vi "Actor Core.vi"(8 "error in":errorcluster, 11 "CS++Motor in":refnum<class "CS++Motor.lvclass">) -> (0 "error out":errorcluster, 3 "Actor out":refnum<class "Actor.lvclass">)   [LabVIEW 2015, in "CS++Motor.lvlib" / "CS++Motor.lvclass"]
doc: "(<B>Filename</B>: Actor Framework.lvlib:Actor.lvclass:Actor Core.vi)\n\nReceives messages to the actor, reacts to them, and initiates any error handling that may shut the actor down.\n\nDescendant classes may override this VI to append parallel tasks for the actor to complete while it handles messages. Overrides use the Call Parent Method node."
uses:
  CS++Motor.lvclass
  <vilib>/ActorFramework/Actor/Actor.lvclass
  CS++Motor.lvclass/CS++Motor.ctl
  <vilib>/ActorFramework/Message Enqueuer/Message Priority.ctl
  <vilib>/ActorFramework/Actor/Actor.lvclass/Actor.ctl
  <vilib>/ActorFramework/Message Enqueuer/Message Enqueuer.lvclass/Message Enqueuer.ctl
  <vilib>/ActorFramework/Report Error Msg/Report Error Msg.lvclass/Report Error Msg.ctl
  <vilib>/ActorFramework/Message Enqueuer/Init from Existing Queue.vi
  <vilib>/ActorFramework/Message Enqueuer/Enqueue.vi
  <vilib>/ActorFramework/Message Priority Queue/Priority Enqueue.vi
  CSPP_Core/Actors/CS++DeviceActor/CS++DeviceActor.lvclass
  <vilib>/ActorFramework/Message Enqueuer/Message Enqueuer.lvclass
  <vilib>/ActorFramework/Report Error Msg/Report Error Msg.lvclass
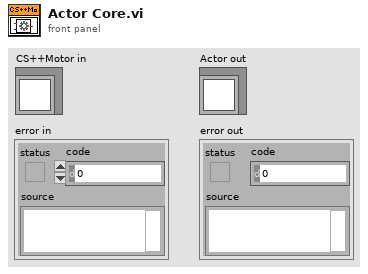
[diagram p1: front panel]
types:
  T1 = typedef "Actor Framework.lvlib/Message Enqueuer.lvclass/Message Priority.ctl" = enum16{"Low", "Normal", "High"}
  T2 = cluster{"AxisNumber":u8, "RawSetPosition":dbl, "Relative?":bool, "RefMove?":bool}[]
  T3 = cluster{"MovementType":enum16{"NormalMovement", "ReferenceMovement", "StopMovement"}, "SetPosition":dbl, "Relative?":bool}
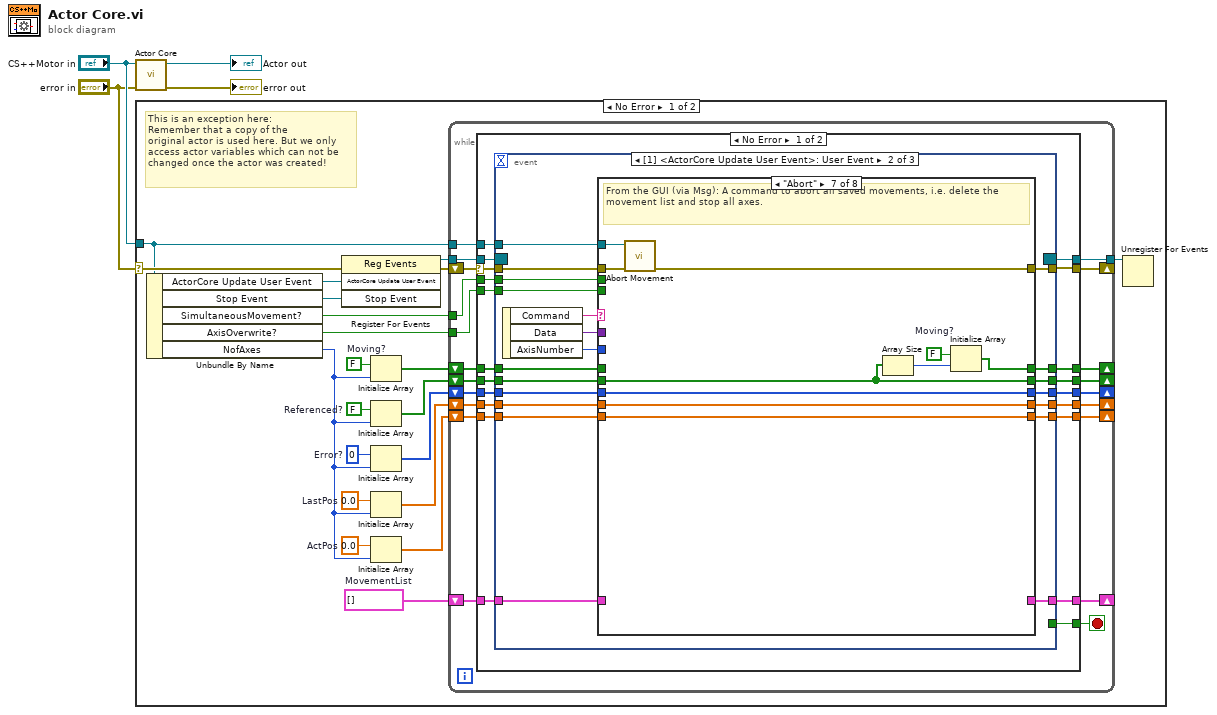
[diagram p0: block diagram]
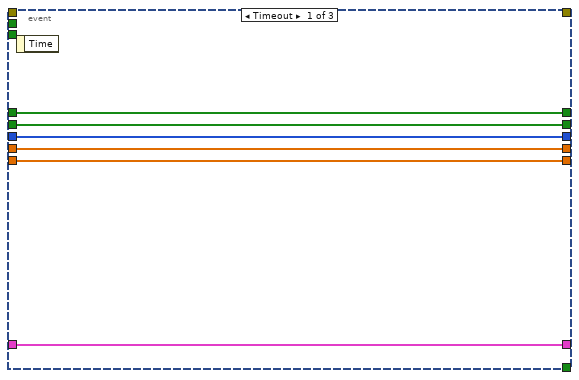
[diagram p2: hidden frame]
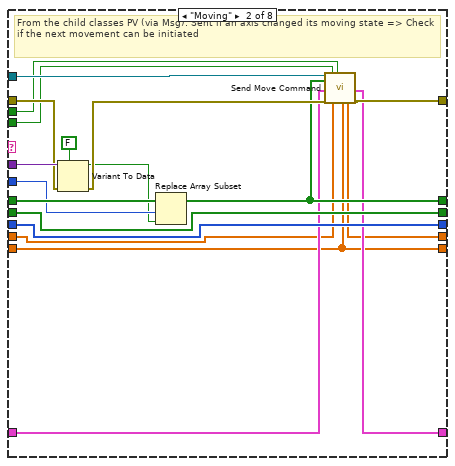
[diagram p4: hidden frame]
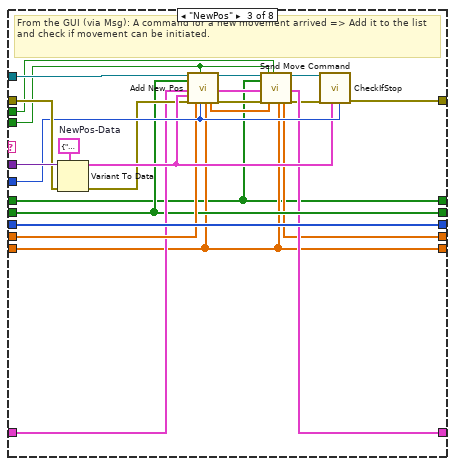
[diagram p5: hidden frame]
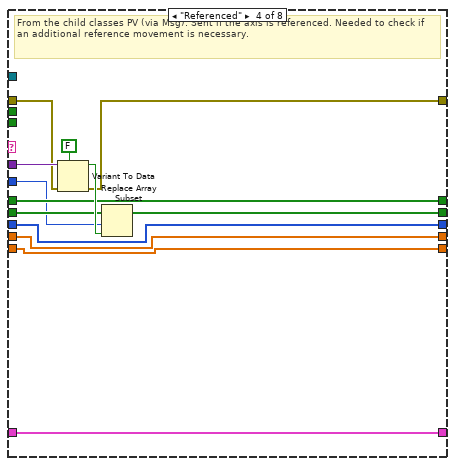
[diagram p6: hidden frame]
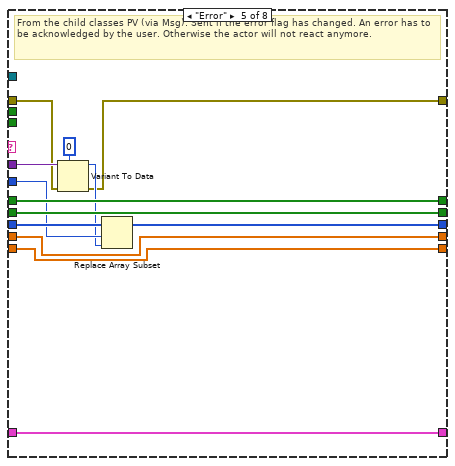
[diagram p7: hidden frame]
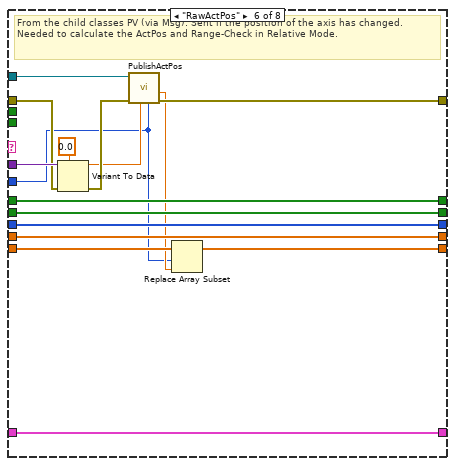
[diagram p8: hidden frame]
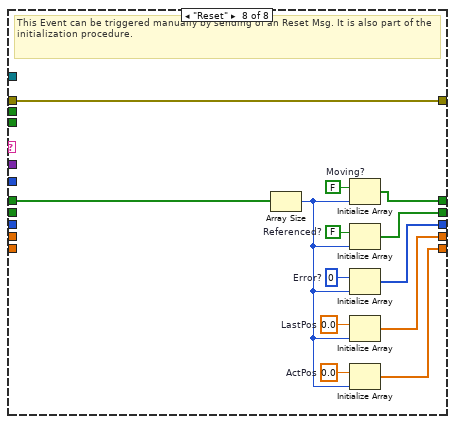
[diagram p9: hidden frame]
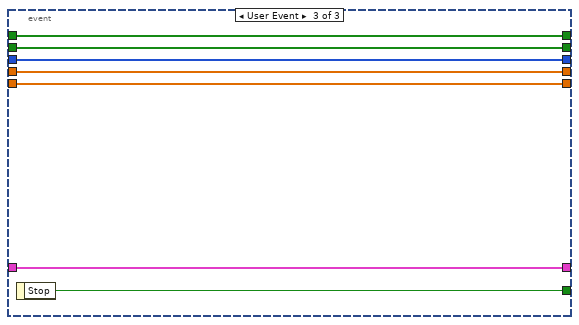
[diagram p10: hidden frame]
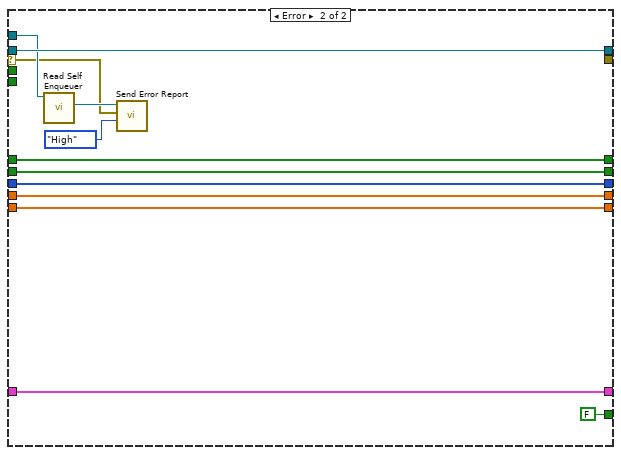
[diagram p11: hidden frame]
diagram:
  n1 = call-parent "Actor Core.vi"("error in"="error in", "CS++BaseActor in"="CS++Motor in") -> ("error out"=→"error out":errorcluster, "Actor out"=→"Actor out":refnum<class "Actor.lvclass">)  [unwired: 8 in]
  n2 = case shown="No Error" "error in" {
    selector: "error in" -> [w15 _]
    tunnel: "CS++Motor in" -> [w13 _]
    frame No Error {
      w9 = 0.0  # ActPos
      w11 = 0.0  # LastPos
      w14 = T2 []  # MovementList
      w20 = i8 0  # Error?
      w22 = FALSE  # Referenced?
      w24 = FALSE  # Moving?
      # "This is an exception here:\nRemember that a copy of the\noriginal actor is used here. But we only\naccess actor variables which can not be\nchanged once the actor was created!"
      n3 = Unbundle By Name(w13) -> ("ActorCore Update User Event"=w17:refnum<user-event>, "Stop Event"=w16:refnum<user-event>, "SimultaneousMovement?"=w7:bool, "AxisOverwrite?"=w6:bool, "NofAxes"=w5:u8)
      n4 = register-events(error in=w15, w17, w16) -> (reference out=w25:refnum<event-registration>, error out=w12:errorcluster)  [unwired: 1 in]
      n5 = Initialize Array(w24, w5) -> (w23:bool[])
      n6 = Initialize Array(w22, w5) -> (w21:bool[])
      n7 = Initialize Array(w20, w5) -> (w19:i8[])
      n8 = Initialize Array(w11, w5) -> (w10:dbl[])
      n9 = Initialize Array(w9, w5) -> (w8:dbl[])
      n10 = while {
        tunnel: w25 -> [w45]
        shift-right: [w41] -> _
        shift-left: w23 -> [w44]
        shift-right: [w39] -> _
        shift-left: w21 -> [w43]
        shift-right: [w40] -> _
        shift-left: w19 -> [w42]
        tunnel: [w38] -> w18
        shift-right: [w33] -> _
        shift-left: w14 -> [w36]
        tunnel: w13 -> [w35]
        tunnel: w7 -> [w34]
        shift-right: [w31] -> _
        shift-left: w12 -> [w32]
        shift-right: [w29] -> _
        shift-left: w10 -> [w30]
        shift-right: [w27] -> _
        shift-left: w8 -> [w28]
        tunnel: w6 -> [w26]
        stop <- w37 stop-if-true
        n11 = case shown="No Error" w32 {
          selector: w32 -> [w52 w217]
          tunnel: w45 -> [w65 w225]
          tunnel: w44 -> [w64 w224]
          tunnel: w43 -> [w63 w223]
          tunnel: w42 -> [w62 w222]
          tunnel: [w61 w224] -> w41
          tunnel: [w60 w222] -> w40
          tunnel: [w59 w223] -> w39
          tunnel: [w58 w225] -> w38
          tunnel: [w57 FALSE] -> w37
          tunnel: w36 -> [w56 w221]
          tunnel: w35 -> [w55 w219]
          tunnel: w34 -> [w54 _]
          tunnel: [w53 w221] -> w33
          tunnel: [w51 _] -> w31
          tunnel: w30 -> [w50 w215]
          tunnel: [w49 w215] -> w29
          tunnel: w28 -> [w48 w214]
          tunnel: [w47 w214] -> w27
          tunnel: w26 -> [w46 _]
          frame No Error {
            n12 = event shown="[1] <ActorCore Update User Event>: User Event" {
              selector: w65 -> [_ _ _]
              dyn-events: [_ _ _] -> w58
              timeout: _ -> [_ _ _]
              tunnel: w64 -> [w68 w90 w213]
              tunnel: w63 -> [w69 w89 w212]
              tunnel: w62 -> [w70 w88 w211]
              tunnel: [w68 w87 w213] -> w61
              tunnel: [w70 w86 w211] -> w60
              tunnel: [w69 w85 w212] -> w59
              tunnel: [_ _ w210] -> w57
              tunnel: w56 -> [w71 w84 w207]
              tunnel: w55 -> [_ w83 _]
              tunnel: w54 -> [_ w81 _]
              tunnel: [w71 w79 w207] -> w53
              tunnel: w52 -> [_ w78 _]
              tunnel: [_ w77 _] -> w51
              tunnel: w50 -> [w67 w76 w209]
              tunnel: [w67 w75 w209] -> w49
              tunnel: w48 -> [w66 w74 w208]
              tunnel: [w66 w73 w208] -> w47
              tunnel: w46 -> [_ w72 _]
              event Timeout {
                n13 = event-data() -> ()  [unwired: 1 in, 1 out]
              }
              event User Event {
                n14 = event-data() -> ("Command"=w91:string, "Data"=w82:variant, "AxisNumber"=w80:u8)  [unwired: 1 in]
                n15 = case shown="\"Abort\"" w91 {
                  tunnel: w90 -> [w98 w117 w118 w149 w166 w182 _ w199]
                  tunnel: w89 -> [w97 w115 w130 w151 w163 w181 w190 _]
                  tunnel: w88 -> [w96 w116 w141 w152 w165 w180 w193 _]
                  tunnel: [w98 w106 w118 w149 w166 w182 w191 w202] -> w87
                  tunnel: [w96 w116 w141 w152 w164 w180 w193 w200] -> w86
                  tunnel: [w97 w115 w130 w150 w163 w181 w190 w201] -> w85
                  tunnel: w84 -> [w94 w103 w131 w144 w157 w174 _ _]
                  tunnel: w83 -> [_ w114 w139 _ _ w177 w186 _]
                  tunnel: w82 -> [_ w113 w140 w148 w162 w179 _ _]
                  tunnel: w81 -> [_ w104 w120 _ _ _ _ _]
                  tunnel: w80 -> [_ w112 w135 w147 w161 w168 _ _]
                  tunnel: [w94 w102 w126 w144 w157 w174 _ _] -> w79
                  tunnel: w78 -> [w95 w111 w137 w146 w159 w178 w185 w206]
                  tunnel: [w95 w107 w136 w145 w158 w175 w184 w206] -> w77
                  tunnel: w76 -> [w93 w101 w133 w143 w156 w172 w188 _]
                  tunnel: [w93 w100 w122 w143 w156 w172 w188 w197] -> w75
                  tunnel: w74 -> [w92 w99 w121 w142 w155 w171 w187 _]
                  tunnel: [w92 w99 w121 w142 w155 w170 w187 w194] -> w73
                  tunnel: w72 -> [_ w105 w119 _ _ _ _ _]
                  frame Default {
                  }
                  frame "Moving" {
                    # "From the child classes PV (via Msg): Sent if an axis changed its moving state => Check if the next movement can be initiated"
                    n16 = Variant To Data(error in=w111, type=FALSE, Variant=w113) -> (data=w108:bool, error out=w110:errorcluster)
                    n17 = Replace Array Subset(array=w117, new element=w108, index=w112) -> (w106:bool[])
                    n18 = call "Send Move Command.vi"("CS++Motor in"=w114, "Moving?"=w106, "MovementList In"=w103, "error in (no error)"=w110, "Axis Overwrite?"=w105, "LastPos In"=w101, "SimultaneousMovement?"=w104, "ActPos"=w99) -> ("LastPos Out"=w100:dbl[], "MovementList Out"=w102:T2, "error out"=w107:errorcluster)  [unwired: 8 in, 1 out]
                  }
                  frame "NewPos" {
                    w138 = T3 {"MovementType"=enum."NormalMovement", "SetPosition"=0.0, "Relative?"=FALSE}  # NewPos-Data
                    # "From the GUI (via Msg): A command for a new movement arrived => Add it to the list and check if movement can be initiated."
                    n19 = Variant To Data(error in=w137, type=w138, Variant=w140) -> (data=w134:T3, error out=w132:errorcluster)
                    n20 = call "Add New Pos.vi"("CS++Motor in"=w139, "Referenced"=w130, "MovementList In"=w131, "NewPos-Data"=w134, "error in (no error)"=w132, "LastPos In"=w133, "Axis Overwrite?"=w119, "AxisNumber"=w135, "ActPos"=w121) -> ("LastPos Out"=w123:dbl[], "CS++Motor out"=w129:refnum<class "CS++Motor.lvclass">, "MovementList Out"=w127:T2, "error out"=w124:errorcluster)  [unwired: 7 in]
                    n21 = call "Send Move Command.vi"("CS++Motor in"=w129, "Moving?"=w118, "MovementList In"=w127, "error in (no error)"=w124, "Axis Overwrite?"=w119, "LastPos In"=w123, "SimultaneousMovement?"=w120, "ActPos"=w121) -> ("LastPos Out"=w122:dbl[], "CS++Motor out"=w128:refnum<class "CS++Motor.lvclass">, "MovementList Out"=w126:T2, "error out"=w125:errorcluster)  [unwired: 8 in]
                    n22 = call "CheckIfStop.vi"("AxisNumber"=w135, "NewPos-Data"=w134, "error in (no error)"=w125, "CS++Motor in"=w128) -> ("error out"=w136:errorcluster)  [unwired: 6 in, 1 out]
                  }
                  frame "Referenced" {
                    # "From the child classes PV (via Msg): Sent if the axis is referenced. Needed to check if an additional reference movement is necessary."
                    n23 = Variant To Data(error in=w146, type=FALSE, Variant=w148) -> (data=w153:bool, error out=w145:errorcluster)
                    n24 = Replace Array Subset(array=w151, new element=w153, index=w147) -> (w150:bool[])
                  }
                  frame "Error" {
                    # "From the child classes PV (via Msg): Sent if the error flag has changed. An error has to be acknowledged by the user. Otherwise the actor will not react anymore."
                    n25 = Variant To Data(error in=w159, type=i8 0, Variant=w162) -> (data=w160:i8, error out=w158:errorcluster)
                    n26 = Replace Array Subset(array=w165, new element=w160, index=w161) -> (w164:i8[])
                  }
                  frame "RawActPos" {
                    # "From the child classes PV (via Msg): Sent if the position of the axis has changed. Needed to calculate the ActPos and Range-Check in Relative Mode."
                    n27 = Variant To Data(error in=w178, type=0.0, Variant=w179) -> (data=w173:dbl, error out=w176:errorcluster)
                    n28 = call "PublishActPos.vi"("AxisNumber"=w168, "RawActPos"=w173, "error in (no error)"=w176, "CS++Motor in"=w177) -> ("error out"=w175:errorcluster, "ActPos"=w169:dbl)  [unwired: 5 in, 1 out]
                    n29 = Replace Array Subset(array=w171, new element=w169, index=w168) -> (w170:dbl[])
                  }
                  frame "Abort" {
                    w192 = FALSE  # Moving?
                    # "From the GUI (via Msg): A command to abort all saved movements, i.e. delete the movement list and stop all axes."
                    n30 = call "Abort Movement.vi"("error in (no error)"=w185, "CS++Motor in"=w186) -> ("error out"=w184:errorcluster)  [unwired: 8 in, 1 out]
                    n31 = Array Size(array=w190) -> (size(s)=w189:i32)
                    n32 = Initialize Array(w192, w189) -> (w191:bool[])
                  }
                  frame "Reset" {
                    w196 = 0.0  # ActPos
                    w198 = 0.0  # LastPos
                    w205 = i8 0  # Error?
                    w204 = FALSE  # Referenced?
                    w203 = FALSE  # Moving?
                    # "This Event can be triggered manually by sending of an Reset Msg. It is also part of the initialization procedure."
                    n33 = Array Size(array=w199) -> (size(s)=w195:i32)
                    n34 = Initialize Array(w203, w195) -> (w202:bool[])
                    n35 = Initialize Array(w204, w195) -> (w201:bool[])
                    n36 = Initialize Array(w205, w195) -> (w200:i8[])
                    n37 = Initialize Array(w198, w195) -> (w197:dbl[])
                    n38 = Initialize Array(w196, w195) -> (w194:dbl[])
                  }
                }
              }
              event User Event {
                n39 = event-data() -> ("Stop"=w210:bool)  [unwired: 1 in]
              }
            }
          }
          frame Error {
            n40 = call <vilib>:"Read Self Enqueuer.vi"("Actor"=w219) -> ("Self Enqueuer"=w218:refnum<class "Message Enqueuer.lvclass">)  [unwired: 10 in]
            n41 = call <vilib>:"Send Error Report.vi"("Message Priority (Normal)"=Message_Priority."High", "Error From Sender"=w217, "Message Enqueuer"=w218) -> ()  [unwired: 8 in, 1 out]
          }
        }
      }
      n42 = Unregister For Events(event registration refnum=w18) -> ()  [unwired: 1 in, 1 out]
    }
    frame Error {
    }
  }
